vi "SetSteeringAngle.vi"(6 "Actuator Channels":T8, 8 "error (in)":errorcluster, 9 "Actuator Active Time":dbl, 10 "Positive?":bool, 11 "Data (in)":T7) -> (0 "error (out)":errorcluster, 2 "Actuator Active Time (out)":dbl, 3 "Data (out)":T7)   [LabVIEW 2015]
doc: "Extend or retract the actuator for the specified amount of time to ensure that the steering angle is reached."
uses:
  <vilib>/MakerHub/LINX/Private/Type Defs/LINX Ref.ctl
  <vilib>/MakerHub/LINX/Private/Type Defs/Platform.ctl
  <vilib>/MakerHub/LINX/Private/Type Defs/Interface.ctl
  <vilib>/MakerHub/LINX/Private/Device/Type Defs/LINX Device Config.ctl
  <vilib>/MakerHub/LINX/Private/Device/Type Defs/TCP Config.ctl
  <vilib>/MakerHub/LINX/Private/Device/Type Defs/Channels.ctl
  <vilib>/MakerHub/LINX/Public/Peripherals/PWM/PWM Set Duty Cycle 1 Chan.vi
  <vilib>/MakerHub/LINX/Public/Peripherals/Digital/Digital Write 1 Chan.vi
  <vilib>/MakerHub/LINX/Public/Peripherals/Digital/Digital Write N Chans.vi
  <vilib>/MakerHub/LINX/Private/Local IO/LinxDigitalWrite.vi
  <vilib>/MakerHub/LINX/Public/Utilities/Check Channel.vi
  <vilib>/MakerHub/LINX/Public/Peripherals/PWM/PWM Set Duty Cycle N Chans.vi
  <vilib>/MakerHub/LINX/Private/Utilties/Generate Error.vi
  <vilib>/MakerHub/LINX/LMH-LINX.lvlib
  <vilib>/MakerHub/LINX/Private/Device/Device.lvlib
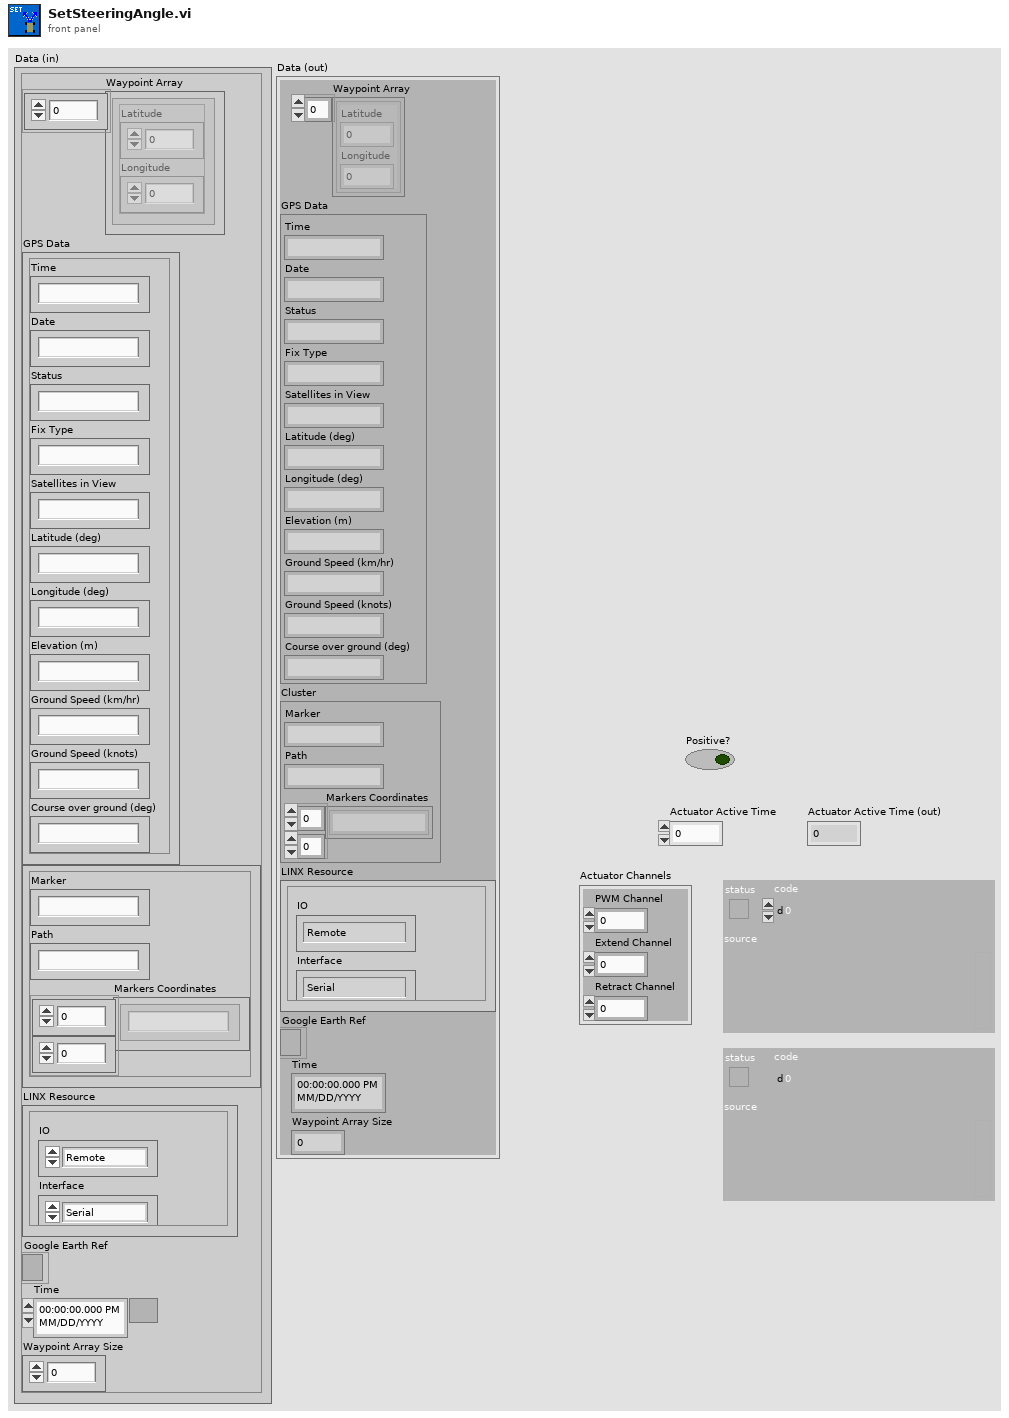
[diagram p1: front panel]
types:
  T1 = typedef "LMH-LINX.lvlib/LINX Ref.ctl" = cluster{"IO":T2, "Interface":T3, "LINX Device Config":T4}
  T2 = typedef "LMH-LINX.lvlib/Platform.ctl" = enum16{"Remote", "Local"}
  T3 = typedef "LMH-LINX.lvlib/Interface.ctl" = enum16{"Serial", "TCP"}
  T4 = typedef "LMH-LINX.lvlib/Device.lvlib/LINX Device Config.ctl" = cluster{"Interface":T3, "COM Port":refnum<visa-resource-name>, "TCP Configuration":T5, "Device Family":u8, "Device ID":u8, "Device Name":string, "TCP Ref":refnum<k5>, "Channels":T6}
  T5 = typedef "LMH-LINX.lvlib/Device.lvlib/TCP Config.ctl" = cluster{"IP Address":string, "Port":u16}
  T6 = typedef "LMH-LINX.lvlib/Channels.ctl" = cluster{"DI":u8[], "DO":u8[], "AI":u8[], "AO":u8[], "PWM":u8[], "QE":u8[], "UART":u8[], "I2C 2":u8[], "SPI":u8[], "CAN":u8[], "Servo":u8[], "AI Ref (V)":dbl, "AI Resolution (Bits)":u8, "AO Ref (V)":dbl, "AO Resolution (Bits)":u8}
  T7 = cluster{"Waypoint Array":cluster{"Latitude":dbl, "Longitude":dbl}[], "GPS Data":cluster{"Time":string, "Date":string, "Status":string, "Fix Type":string, "Satellites in View":string, "Latitude (deg)":string, "Longitude (deg)":string, "Elevation (m)":string, "Ground Speed (km/hr)":string, "Ground Speed (knots)":string, "Course over ground (deg)":string}, "Cluster":cluster{"Marker":string, "Path":string, "Markers Coordinates":string[][]}, "LINX Resource":T1, "Google Earth Ref":refnum<k7>, "Time":timestamp, "Waypoint Array Size":i32}
  T8 = cluster{"PWM Channel":u8, "Extend Channel":u8, "Retract Channel":u8}
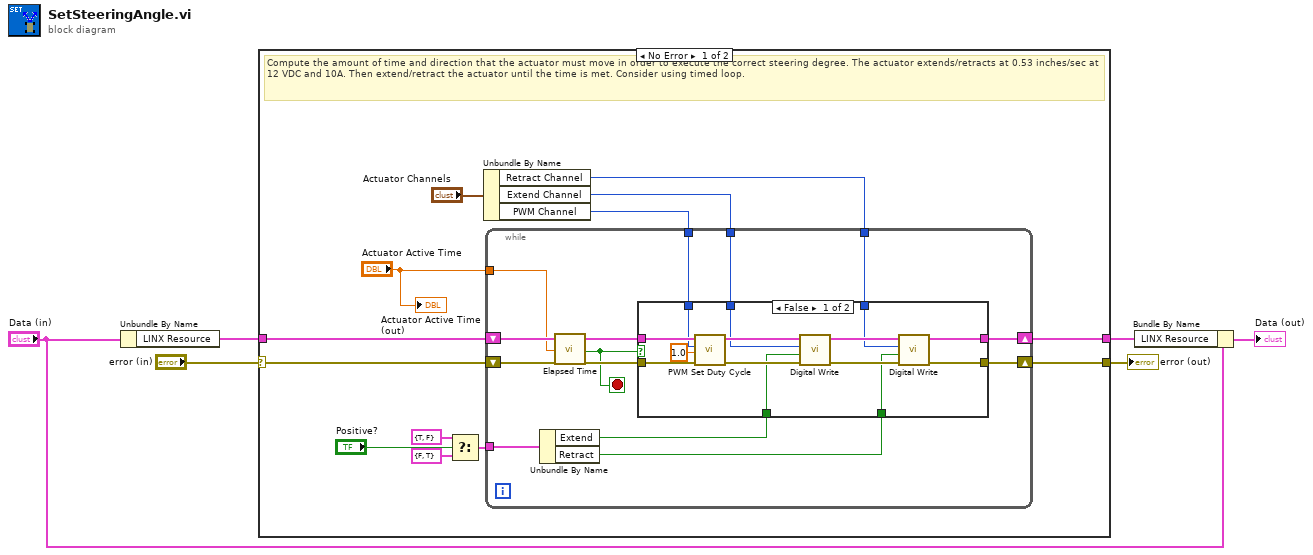
[diagram p0: block diagram]
diagram:
  n1 = Unbundle By Name("Data (in)") -> ("LINX Resource"=w4:T1)
  n2 = case shown="No Error" "error (in)" {
    selector: "error (in)" -> [w17 w50]
    tunnel: [w13 w50] -> w5
    tunnel: w4 -> [w19 w49]
    tunnel: [w18 w49] -> w3
    frame No Error {
      # "Compute the amount of time and direction that the actuator must move in order to execute the correct steering degree. The actuator extends/retracts at 0.53 inches/sec at 12 VDC and 10A. Then extend/retract the actuator until the time is met. Consider using timed loop."
      n3 = Select(t=cluster{"Extend":bool, "Retract":bool} {"Extend"=TRUE, "Retract"=FALSE}, s="Positive?", f=cluster{"Extend":bool, "Retract":bool} {"Extend"=FALSE, "Retract"=TRUE}) -> (s? t:f=w14:cluster{"Extend":bool, "Retract":bool})
      n4 = Unbundle By Name("Actuator Channels") -> ("Retract Channel"=w11:u8, "Extend Channel"=w10:u8, "PWM Channel"=w9:u8)
      n5 = while {
        shift-right: [w30] -> w18
        shift-left: w19 -> [w32]
        shift-right: [w29] -> w13
        shift-left: w17 -> [w23]
        tunnel: w14 -> [w31]
        tunnel: w11 -> [w26]
        tunnel: w10 -> [w27]
        tunnel: w9 -> [w28]
        tunnel: "Actuator Active Time" -> [w21]
        stop <- w20 stop-if-true
        n6 = Unbundle By Name(w31) -> ("Extend"=w25:bool, "Retract"=w24:bool)
        n7 = call "Elapsed Time"("Time Target (s)"=w21, "error in (no error)"=w23) -> ("Time has Elapsed"=w20:bool, "error out"=w22:errorcluster)  [unwired: 10 in, 6 out]
        n8 = case shown="False" w20 {
          tunnel: w22 -> [w42 w47]
          tunnel: w32 -> [w41 w48]
          tunnel: w24 -> [w40 _]
          tunnel: w25 -> [w39 _]
          tunnel: [w38 w48] -> w30
          tunnel: [w37 w47] -> w29
          tunnel: w28 -> [w35 _]
          tunnel: w27 -> [w34 _]
          tunnel: w26 -> [w33 _]
          frame False {
            n9 = call-poly <vilib>:"PWM Set Duty Cycle.vi"("Error In"=w42, "Duty Cycle (0-1)"=1.0, "PWM Channel"=w35, "LINX Resource"=w41) -> ("Error Out"=w45:errorcluster, "LINX Resource"=w46:T1)  [unwired: 6 in]
            n10 = call-poly <vilib>:"Digital Write.vi"("Error In"=w45, "Output Value"=w39, "DO Channel"=w34, "LINX Resource"=w46) -> ("Error Out"=w44:errorcluster, "LINX Resource"=w43:T1)  [unwired: 6 in]
            n11 = call-poly <vilib>:"Digital Write.vi"("Error In"=w44, "Output Value"=w40, "DO Channel"=w33, "LINX Resource"=w43) -> ("Error Out"=w37:errorcluster, "LINX Resource"=w38:T1)  [unwired: 6 in]
          }
          frame True {
          }
        }
      }
      "Actuator Active Time (out)" <- "Actuator Active Time"
    }
    frame Error {
      # "error has occured - pass error through case structure"
    }
  }
  "error (out)" <- w5
  n12 = Bundle By Name(cluster="Data (in)", "LINX Resource"=w3) -> (→"Data (out)":T7)
